vi "Flipper Delay Test.vi"() -> ()   [LabVIEW 2012]
panel:
  in  "Shoot Mode":bool
  in  "Shoot Button":bool
  in  "Shooting Delays":T1={"Unjam On"=100.0, "Unjam Off"=100.0, "Flipper On"=300.0, "Flipper Off"=200.0, "Hopper Up"=100.0}
  in  "milliseconds to wait":u32=1000
  out "Processing":bool=TRUE
  out "Unjam Out":bool
  out "Flipper Out":bool
  in  "RPM In Range":bool
  in  "stop":bool
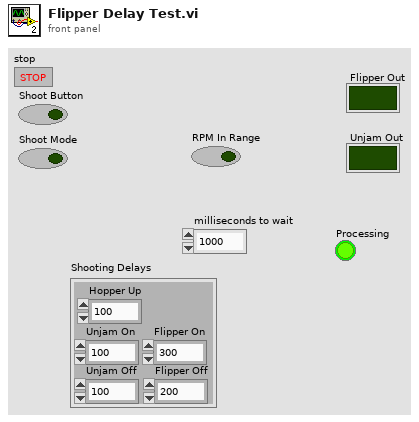
[diagram p1: front panel]
types:
  T1 = cluster{"Unjam On":dbl, "Unjam Off":dbl, "Flipper On":dbl, "Flipper Off":dbl, "Hopper Up":dbl}
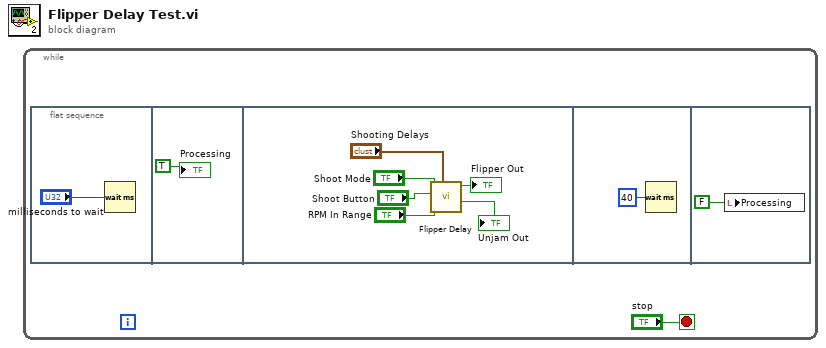
[diagram p0: block diagram]
diagram:
  n1 = while {
    stop <- "stop" stop-if-true
    n2 = flat-sequence {
      frame #0 {
        n3 = Wait (ms)(milliseconds to wait="milliseconds to wait") -> ()  [unwired: 1 out]
      }
      frame #1 {
        "Processing" <- TRUE
      }
      frame #2 {
        n4 = call "Flipper Delay.vi"("Shooting Delays"="Shooting Delays", "RPM In Range"="RPM In Range", "Shoot Button"="Shoot Button", "Shoot Mode"="Shoot Mode") -> ("Unjam Out"=→"Unjam Out":bool, "Flipper Out"=→"Flipper Out":bool)  [unwired: 6 in]
      }
      frame #3 {
        n5 = Wait (ms)(milliseconds to wait=u32 40) -> ()  [unwired: 1 out]
      }
      frame #4 {
        n6 = local write "Processing"(FALSE ("Processing")) -> ()
      }
    }
  }
